vi "Kinesis-Microestruturacao-Circuits.vi"() -> ()   [LabVIEW 2014]
doc: "André Romero - 2017\nandretec@ifsc.usp.br"
uses:
  Basic-VIs/motorsGlobalVar.vi
  <vilib>/Instr/_visa.llb/VISA Configure Serial Port (Instr).vi
  C:/user-Lab/AndreTec/GITs/andretec/Thorlabs-Vector-Move/kinesisTec/Kinesis/Thorlabs.MotionControl.Controls.dll
  kinesisTec/Kinesis/Thorlabs.MotionControl.Controls.dll
panel:
  in  "Raio":dbl=0.01
  in  "Density":dbl=100.0
  in  "Adjust Motors":bool
  out "Process time":string="0:00:50"
  out "Progress %":dbl(slide) scale=0.0..100.0
  out "XY Graph":cluster{"Graph X":dbl[], "Graph Y":dbl[]}(graph)
  in  "Swap XY":bool
  out "stop cronometro":bool=TRUE
  in  "Stop Button":bool
  in  "Graph Y":dbl[](array[numeric])=[0.0, 0.0, 6.6674440298507465, 6.6674440298507465, 6.6674440298507465, 6.6674440298507465, 6.6674440298507465, 6.6674440298507465, 6.6674440298507465, 6.6674440298507465, 6.6674440298507465, 6.6674440298507465, 6.6674440298507465, 6.6674440298507465, 6.6674440298507465, 6.6674440298507465, 6.6674440298507465, 6.6674440298507465, 6.6674440298507465, 6.6674440298507465, 6.6674440298507465, 6.6674440298507465, 6.6674440298507465, 6.6674440298507465, 6.6674440298507465, 6.6674440298507465, 6.6674440298507465, 6.6674440298507465, 6.6674440298507465, 6.6674440298507465, 6.6674440298507465, 6.6674440298507465, 6.6674440298507465, 6.6674440298507465, 6.6674440298507465, 6.6674440298507465, 6.6674440298507465, 6.6674440298507465, 6.6674440298507465, 6.6674440298507465, 6.6674440298507465, 6.6674440298507465, 6.6674440298507465, 6.673128498134329, 6.673128498134329, 6.673128498134329, 6.673128498134329, 6.673128498134329, 6.687354244402985, 6.687354244402985, 6.687354244402985, 6.687354244402985, 6.687354244402985, 6.692543143656716, 6.692543143656716, 6.692543143656716, 6.692543143656716, 6.692543143656716, 6.692543143656716, 6.692543143656716, 6.692543143656716, 6.692543143656716, 6.692543143656716, 6.692543143656716, 6.692543143656716, 6.691522854477612, 6.691522854477612, 6.691522854477612, 6.691522854477612, 6.691522854477612, 6.680183069029851, 6.680183069029851, 6.680183069029851, 6.680183069029851, 6.680183069029851, 6.658640391791045, 6.658640391791045, 6.658640391791045, 6.658640391791045, 6.658640391791045, 6.644793610074627, 6.644793610074627, 6.644793610074627, 6.644793610074627, 6.644793610074627, 6.642490671641791, 6.642490671641791, 6.642490671641791, 6.642490671641791, 6.642490671641791, 6.642490671641791, 6.642490671641791, 6.642490671641791, 6.642490671641791, 6.642490671641791, 6.642490671641791, 6.642490671641791, 6.642490671641791, 6.642490671641791, 6.642490671641791, 6.647825326492537, 6.647825326492537, 6.647825326492537, 6.647825326492537, 6.647825326492537, 6.66543260261194, 6.66543260261194, 6.66543260261194, 6.66543260261194, 6.66543260261194, 6.685226212686567, 6.685226212686567, 6.685226212686567, 6.685226212686567, 6.685226212686567, 6.692484841417911, 6.692484841417911, 6.692484841417911, 6.692484841417911, 6.692484841417911, 6.692543143656716, 6.692543143656716, 6.692543143656716, 6.692543143656716, 6.692543143656716, 6.692543143656716, 6.692543143656716, 6.691464552238806, 6.691464552238806, 6.691464552238806, 6.691464552238806, 6.691464552238806, 6.679833255597015, 6.679833255597015, 6.679833255597015, 6.679833255597015, 6.679833255597015, 6.658057369402985, 6.658057369402985, 6.658057369402985, 6.658057369402985, 6.658057369402985, 6.644647854477612, 6.644647854477612, 6.644647854477612, 6.644647854477612, 6.644647854477612, 6.642548973880597, 6.642548973880597, 6.642548973880597, 6.642548973880597, 6.642548973880597, 6.642519822761194, 6.642519822761194, 6.642519822761194, 6.642519822761194, 6.642519822761194, 6.642519822761194, 6.642519822761194, 6.642519822761194, 6.643569263059701, 6.643569263059701, 6.643569263059701, 6.643569263059701, 6.643569263059701, 6.655521222014926, 6.655521222014926, 6.655521222014926, 6.655521222014926, 6.655521222014926, 6.677180503731344, 6.677180503731344, 6.677180503731344, 6.677180503731344, 6.677180503731344, 6.690531716417911, 6.690531716417911, 6.690531716417911, 6.690531716417911, 6.690531716417911, 6.692572294776119, 6.692572294776119, 6.692572294776119, 6.692572294776119, 6.692572294776119, 6.692572294776119, 6.692572294776119, 6.692572294776119, 6.692572294776119, 6.692572294776119, 6.692572294776119, 6.692572294776119, 6.691522854477612, 6.691522854477612, 6.691522854477612, 6.691522854477612, 6.691522854477612, 6.680008162313433, 6.680008162313433, 6.680008162313433, 6.680008162313433, 6.680008162313433, 6.668668376865671, 6.668668376865671, 6.668668376865671, 6.668668376865671, 6.668668376865671, 6.667502332089552, 6.667502332089552, 6.667502332089552, 6.667502332089552, 6.667502332089552, 6.667502332089552, 6.667502332089552, 6.667502332089552, 6.667502332089552, 6.667502332089552, 6.667502332089552, 6.667502332089552, 6.667531483208955, 6.667531483208955, 6.667531483208955, 6.667531483208955, 6.667531483208955, 6.667531483208955, 6.667531483208955, 6.667531483208955, 6.667531483208955, 6.667531483208955, 6.667531483208955, 6.667531483208955, 6.667531483208955, 6.667531483208955, 6.667531483208955, 6.667531483208955, 6.667531483208955, 6.667531483208955, 6.667531483208955, 6.667531483208955, 6.667531483208955, 6.667531483208955, 6.667531483208955, 6.667531483208955, 6.667531483208955, 6.667531483208955, 6.667531483208955, 6.667531483208955, 6.667531483208955, 6.667531483208955, 6.667531483208955, 6.667531483208955, 6.667531483208955, 6.667531483208955, 6.667531483208955, 6.667531483208955, 6.667531483208955, 6.6663945895522385, 6.6663945895522385, 6.6663945895522385, 6.6663945895522385, 6.6663945895522385, 6.662051072761194, 6.662051072761194, 6.662051072761194, 6.662051072761194, 6.662051072761194, 6.644035680970149, 6.644035680970149, 6.644035680970149, 6.644035680970149, 6.644035680970149, 6.606430736940299, 6.606430736940299, 6.606430736940299, 6.606430736940299, 6.606430736940299, 6.593924906716418, 6.593924906716418, 6.593924906716418, 6.593924906716418, 6.593924906716418, 6.574539412313433, 6.574539412313433, 6.574539412313433, 6.574539412313433, 6.574539412313433, 6.567484841417911, 6.567484841417911, 6.567484841417911, 6.567484841417911, 6.567484841417911, 6.567484841417911, 6.567484841417911, 6.567484841417911, 6.567484841417911, 6.567484841417911, 6.567484841417911, 6.567513992537314, 6.567513992537314, 6.567513992537314, 6.567513992537314, 6.567513992537314, 6.567513992537314, 6.567513992537314, 6.567513992537314, 6.567513992537314, 6.567513992537314, 6.567543143656716, 6.567543143656716, 6.567543143656716, 6.567543143656716, 6.567543143656716, 6.567543143656716, 6.567543143656716, 6.567543143656716, 6.567543143656716, 6.567543143656716, 6.567543143656716, 6.567543143656716, 6.567543143656716, 6.567543143656716, 6.567543143656716, 6.567543143656716, 6.567543143656716, 6.567543143656716, 6.567543143656716, 6.567543143656716, 6.567543143656716, 6.567543143656716, 6.567543143656716, 6.567543143656716, 6.567543143656716, 6.567543143656716, 6.567543143656716, 6.567543143656716, 6.567543143656716, 6.567543143656716, 6.567543143656716, 6.567543143656716, 6.567543143656716, 6.567543143656716, 6.567543143656716, 6.567543143656716, 6.567543143656716, 6.567543143656716, 6.567543143656716, 6.567543143656716, 6.567543143656716, 6.567543143656716, 6.567543143656716, 6.567543143656716, 6.567543143656716, 6.567543143656716, 6.567543143656716, 6.567543143656716, 6.567543143656716, 6.567543143656716, 6.567543143656716, 6.567543143656716, 6.567543143656716, 6.567543143656716, 6.5667852145522385, 6.5667852145522385, 6.5667852145522385, 6.5667852145522385, 6.5667852145522385, 6.555299673507463, 6.555299673507463, 6.555299673507463, 6.555299673507463, 6.555299673507463, 6.533523787313433, 6.533523787313433, 6.533523787313433, 6.533523787313433, 6.533523787313433, 6.525186567164179, 6.525186567164179, 6.525186567164179, 6.525186567164179, 6.525186567164179, 6.517490671641791, 6.517490671641791, 6.517490671641791, 6.517490671641791, 6.517490671641791, 6.517490671641791, 6.517490671641791, 6.517490671641791, 6.517490671641791, 6.517490671641791, 6.517519822761194, 6.517519822761194, 6.517519822761194, 6.517519822761194, 6.517519822761194, 6.517519822761194, 6.517519822761194, 6.517519822761194, 6.517519822761194, 6.517519822761194, 6.517548973880597, 6.517548973880597, 6.517548973880597, 6.517548973880597, 6.517548973880597, 6.517548973880597, 6.517548973880597, 6.517548973880597, 6.517548973880597, 6.517548973880597, 6.517548973880597, 6.517548973880597, 6.517548973880597, 6.517548973880597, 6.517548973880597, 6.517548973880597, 6.517548973880597, 6.517548973880597, 6.517548973880597, 6.517548973880597, 6.517548973880597, 6.517548973880597, 6.517548973880597, 6.517548973880597, 6.517548973880597, 6.517548973880597, 6.517548973880597, 6.517548973880597, 6.517548973880597, 6.517548973880597, 6.517548973880597, 6.517548973880597, 6.517548973880597, 6.517548973880597, 6.517548973880597, 6.517548973880597, 6.517548973880597, 6.517548973880597, 6.517548973880597, 6.517548973880597, 6.517548973880597, 6.517548973880597, 6.517548973880597, 6.517548973880597, 6.517548973880597, 6.517548973880597, 6.517548973880597, 6.517548973880597, 6.517548973880597, 6.517548973880597, 6.517548973880597, 6.517548973880597, 6.517548973880597, 6.517548973880597, 6.517548973880597, 6.517548973880597, 6.517548973880597, 6.517548973880597, 6.517548973880597, 6.517548973880597, 6.516674440298507, 6.516674440298507, 6.516674440298507, 6.516674440298507, 6.516674440298507, 6.504897388059701, 6.504897388059701, 6.504897388059701, 6.504897388059701, 6.504897388059701, 6.481926305970149, 6.481926305970149, 6.481926305970149, 6.481926305970149, 6.481926305970149, 6.456943796641791, 6.456943796641791, 6.456943796641791, 6.456943796641791, 6.456943796641791, 6.4330690298507465, 6.4330690298507465, 6.4330690298507465, 6.4330690298507465, 6.4330690298507465, 6.419717817164179, 6.419717817164179, 6.419717817164179, 6.419717817164179, 6.419717817164179, 6.417473180970149, 6.417473180970149, 6.417473180970149, 6.417473180970149, 6.417473180970149, 6.417473180970149]
  in  "Graph X":dbl[](array[numeric])=[0.0, 0.0, 3.605935167910448, 3.605935167910448, 3.605935167910448, 3.605935167910448, 3.605935167910448, 3.609987173507463, 3.609987173507463, 3.609987173507463, 3.609987173507463, 3.609987173507463, 3.627157182835821, 3.627157182835821, 3.627157182835821, 3.627157182835821, 3.627157182835821, 3.6520813899253732, 3.6520813899253732, 3.6520813899253732, 3.6520813899253732, 3.6520813899253732, 3.6770930503731343, 3.6770930503731343, 3.6770930503731343, 3.6770930503731343, 3.6770930503731343, 3.697323927238806, 3.697323927238806, 3.697323927238806, 3.697323927238806, 3.697323927238806, 3.705311333955224, 3.705311333955224, 3.705311333955224, 3.705311333955224, 3.705311333955224, 3.705311333955224, 3.705311333955224, 3.705311333955224, 3.705311333955224, 3.705311333955224, 3.705311333955224, 3.7063024720149254, 3.7063024720149254, 3.7063024720149254, 3.7063024720149254, 3.7063024720149254, 3.7175839552238807, 3.7175839552238807, 3.7175839552238807, 3.7175839552238807, 3.7175839552238807, 3.7291861007462686, 3.7291861007462686, 3.7291861007462686, 3.7291861007462686, 3.7291861007462686, 3.7303521455223883, 3.7303521455223883, 3.7303521455223883, 3.7303521455223883, 3.7303521455223883, 3.7303521455223883, 3.7303521455223883, 3.7303521455223883, 3.7303521455223883, 3.7303521455223883, 3.7303521455223883, 3.7303521455223883, 3.7366779384328357, 3.7366779384328357, 3.7366779384328357, 3.7366779384328357, 3.7366779384328357, 3.7554221082089554, 3.7554221082089554, 3.7554221082089554, 3.7554221082089554, 3.7554221082089554, 3.774137126865672, 3.774137126865672, 3.774137126865672, 3.774137126865672, 3.774137126865672, 3.7803463152985075, 3.7803463152985075, 3.7803463152985075, 3.7803463152985075, 3.7803463152985075, 3.7803463152985075, 3.7803463152985075, 3.7803463152985075, 3.7803463152985075, 3.7803463152985075, 3.7803463152985075, 3.7803463152985075, 3.7803463152985075, 3.7803463152985075, 3.7803463152985075, 3.781803871268657, 3.781803871268657, 3.781803871268657, 3.781803871268657, 3.781803871268657, 3.7941930970149254, 3.7941930970149254, 3.7941930970149254, 3.7941930970149254, 3.7941930970149254, 3.816027285447761, 3.816027285447761, 3.816027285447761, 3.816027285447761, 3.816027285447761, 3.828678871268657, 3.828678871268657, 3.828678871268657, 3.828678871268657, 3.828678871268657, 3.8303404850746268, 3.8303404850746268, 3.8303404850746268, 3.8303404850746268, 3.8303404850746268, 3.8303404850746268, 3.8303404850746268, 3.8303404850746268, 3.8303404850746268, 3.8303404850746268, 3.8303404850746268, 3.8303404850746268, 3.8368703358208953, 3.8368703358208953, 3.8368703358208953, 3.8368703358208953, 3.8368703358208953, 3.8447994402985075, 3.8447994402985075, 3.8447994402985075, 3.8447994402985075, 3.8447994402985075, 3.866633628731343, 3.866633628731343, 3.866633628731343, 3.866633628731343, 3.866633628731343, 3.8803346548507465, 3.8803346548507465, 3.8803346548507465, 3.8803346548507465, 3.8803346548507465, 3.8803346548507465, 3.8803346548507465, 3.8803346548507465, 3.8803346548507465, 3.8803346548507465, 3.8803346548507465, 3.8803346548507465, 3.8803346548507465, 3.8803346548507465, 3.8803346548507465, 3.8803346548507465, 3.8803346548507465, 3.8803346548507465, 3.886631296641791, 3.886631296641791, 3.886631296641791, 3.886631296641791, 3.886631296641791, 3.9054046175373136, 3.9054046175373136, 3.9054046175373136, 3.9054046175373136, 3.9054046175373136, 3.92411963619403, 3.92411963619403, 3.92411963619403, 3.92411963619403, 3.92411963619403, 3.9303288246268657, 3.9303288246268657, 3.9303288246268657, 3.9303288246268657, 3.9303288246268657, 3.9303288246268657, 3.9303288246268657, 3.9303288246268657, 3.9303288246268657, 3.9303288246268657, 3.9303288246268657, 3.9303288246268657, 3.9303288246268657, 3.9303288246268657, 3.9303288246268657, 3.9303288246268657, 3.9303288246268657, 3.936800373134328, 3.936800373134328, 3.936800373134328, 3.936800373134328, 3.936800373134328, 3.9445545708955225, 3.9445545708955225, 3.9445545708955225, 3.9445545708955225, 3.9445545708955225, 3.95536963619403, 3.95536963619403, 3.95536963619403, 3.95536963619403, 3.95536963619403, 3.95536963619403, 3.95536963619403, 3.95536963619403, 3.95536963619403, 3.95536963619403, 3.95536963619403, 3.95536963619403, 3.956652285447761, 3.956652285447761, 3.956652285447761, 3.956652285447761, 3.956652285447761, 3.961141557835821, 3.961141557835821, 3.961141557835821, 3.961141557835821, 3.961141557835821, 3.9795067630597014, 3.9795067630597014, 3.9795067630597014, 3.9795067630597014, 3.9795067630597014, 4.004518423507463, 4.004518423507463, 4.004518423507463, 4.004518423507463, 4.004518423507463, 4.0406366604477615, 4.0406366604477615, 4.0406366604477615, 4.0406366604477615, 4.0406366604477615, 4.048624067164179, 4.048624067164179, 4.048624067164179, 4.048624067164179, 4.048624067164179, 4.0553579757462686, 4.0553579757462686, 4.0553579757462686, 4.0553579757462686, 4.0553579757462686, 4.0553579757462686, 4.0553579757462686, 4.055387126865671, 4.055387126865671, 4.055387126865671, 4.055387126865671, 4.055387126865671, 4.055387126865671, 4.055387126865671, 4.055387126865671, 4.055387126865671, 4.055387126865671, 4.0553579757462686, 4.0553579757462686, 4.0553579757462686, 4.0553579757462686, 4.0553579757462686, 4.0553579757462686, 4.0553579757462686, 4.0553579757462686, 4.0553579757462686, 4.0553579757462686, 4.0553579757462686, 4.0553579757462686, 4.0553579757462686, 4.0553579757462686, 4.0553579757462686, 4.0553579757462686, 4.0553579757462686, 4.0553579757462686, 4.0553579757462686, 4.0553579757462686, 4.0553579757462686, 4.0553579757462686, 4.0553579757462686, 4.0553579757462686, 4.0553579757462686, 4.0553579757462686, 4.0553579757462686, 4.0553579757462686, 4.0553579757462686, 4.0553579757462686, 4.0553579757462686, 4.061800373134329, 4.061800373134329, 4.061800373134329, 4.061800373134329, 4.061800373134329, 4.06972947761194, 4.06972947761194, 4.06972947761194, 4.06972947761194, 4.06972947761194, 4.091534514925373, 4.091534514925373, 4.091534514925373, 4.091534514925373, 4.091534514925373, 4.105352145522388, 4.105352145522388, 4.105352145522388, 4.105352145522388, 4.105352145522388, 4.105381296641791, 4.105381296641791, 4.105381296641791, 4.105381296641791, 4.105381296641791, 4.105381296641791, 4.105381296641791, 4.1050897854477615, 4.1050897854477615, 4.1050897854477615, 4.1050897854477615, 4.1050897854477615, 4.0951784048507465, 4.0951784048507465, 4.0951784048507465, 4.0951784048507465, 4.0951784048507465, 4.073489972014926, 4.073489972014926, 4.073489972014926, 4.073489972014926, 4.073489972014926, 4.060954990671642, 4.060954990671642, 4.060954990671642, 4.060954990671642, 4.060954990671642, 4.023874766791045, 4.023874766791045, 4.023874766791045, 4.023874766791045, 4.023874766791045, 4.008687033582089, 4.008687033582089, 4.008687033582089, 4.008687033582089, 4.008687033582089, 4.005363805970149, 4.005363805970149, 4.005363805970149, 4.005363805970149, 4.005363805970149, 4.005363805970149, 4.005363805970149, 4.005363805970149, 4.005363805970149, 4.005363805970149, 4.005363805970149, 4.005363805970149, 4.005363805970149, 4.005363805970149, 4.005363805970149, 4.005363805970149, 4.005363805970149, 4.005392957089552, 4.005392957089552, 4.005392957089552, 4.005392957089552, 4.005392957089552, 4.005392957089552, 4.005392957089552, 4.005392957089552, 4.005392957089552, 4.005392957089552, 4.005392957089552, 4.005392957089552, 4.005392957089552, 4.005392957089552, 4.005392957089552, 4.005392957089552, 4.005392957089552, 4.005392957089552, 4.005392957089552, 4.005392957089552, 4.011631296641791, 4.011631296641791, 4.011631296641791, 4.011631296641791, 4.011631296641791, 4.019472947761194, 4.019472947761194, 4.019472947761194, 4.019472947761194, 4.019472947761194, 4.042852145522388, 4.042852145522388, 4.042852145522388, 4.042852145522388, 4.042852145522388, 4.080398787313433, 4.080398787313433, 4.080398787313433, 4.080398787313433, 4.080398787313433, 4.099113805970149, 4.099113805970149, 4.099113805970149, 4.099113805970149, 4.099113805970149, 4.103777985074627, 4.103777985074627, 4.103777985074627, 4.103777985074627, 4.103777985074627, 4.105410447761194, 4.105410447761194, 4.105410447761194, 4.105410447761194, 4.105410447761194, 4.105410447761194, 4.105410447761194, 4.105410447761194, 4.105381296641791, 4.105381296641791, 4.105381296641791, 4.105381296641791, 4.105381296641791, 4.098297574626866, 4.098297574626866, 4.098297574626866, 4.098297574626866, 4.098297574626866, 4.089989505597015, 4.089989505597015, 4.089989505597015, 4.089989505597015, 4.089989505597015, 4.06083838619403, 4.06083838619403, 4.06083838619403, 4.06083838619403, 4.06083838619403, 4.0553579757462686, 4.0553579757462686, 4.0553579757462686, 4.0553579757462686, 4.0553579757462686, 4.0553579757462686, 4.0553579757462686, 4.0553579757462686, 4.0553579757462686, 4.0553579757462686, 4.0553579757462686, 4.0553579757462686, 4.055387126865671, 4.055387126865671, 4.055387126865671, 4.055387126865671, 4.055387126865671, 4.055416277985074, 4.055416277985074, 4.055416277985074, 4.055416277985074, 4.055416277985074, 4.055416277985074, 4.055416277985074, 4.055416277985074, 4.055416277985074, 4.055416277985074, 4.055416277985074, 4.055416277985074, 4.055416277985074, 4.055416277985074, 4.055416277985074, 4.055416277985074, 4.055416277985074, 4.055416277985074, 4.055416277985074, 4.055416277985074, 4.055416277985074, 4.055416277985074, 4.055416277985074, 4.055416277985074, 4.055416277985074, 4.055416277985074, 4.055416277985074, 4.055416277985074, 4.055416277985074, 4.055416277985074, 4.055416277985074]
  out "GetPOS Y":dbl=6.417473180970149 format="%_6f"
  out "GetPOS X":dbl=4.055416277985074 format="%#_6f"
  out ".NET Refnum out 2":refnum<k24>
  out ".NET Refnum out 1":refnum<k24>
  out "Motor 2":bool
  out "Motor 1":bool
  in  "Acceleration (mm/s)":dbl=0.05
  in  "Iniciar":bool
  in  "Velocity (mm/s)":sgl=0.05
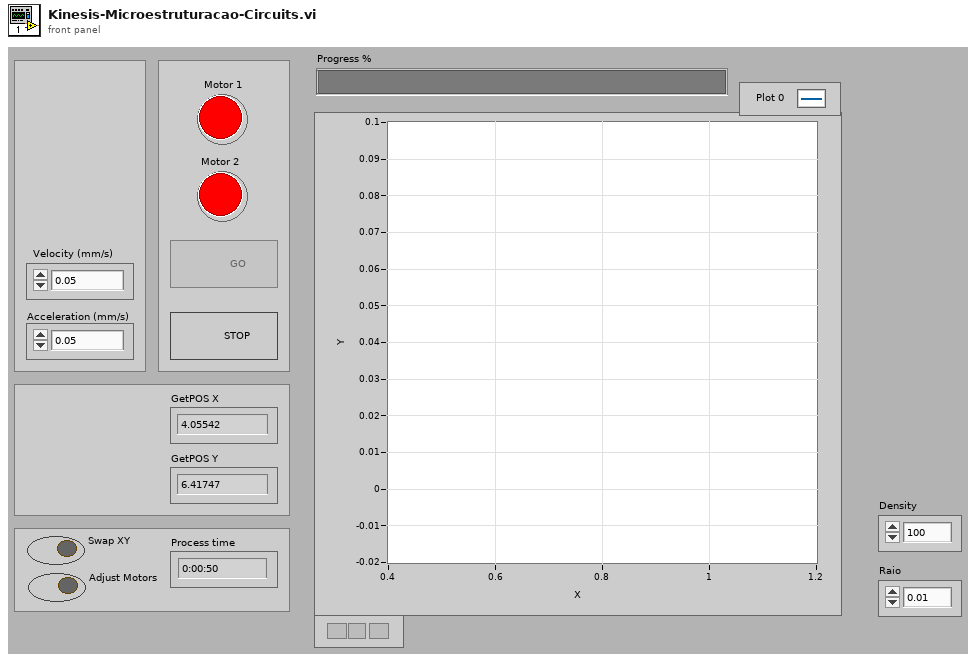
[diagram p1: front panel]
types:
  T1 = enum8{"Enabled", "Disabled", "Disabled and Grayed Out"}
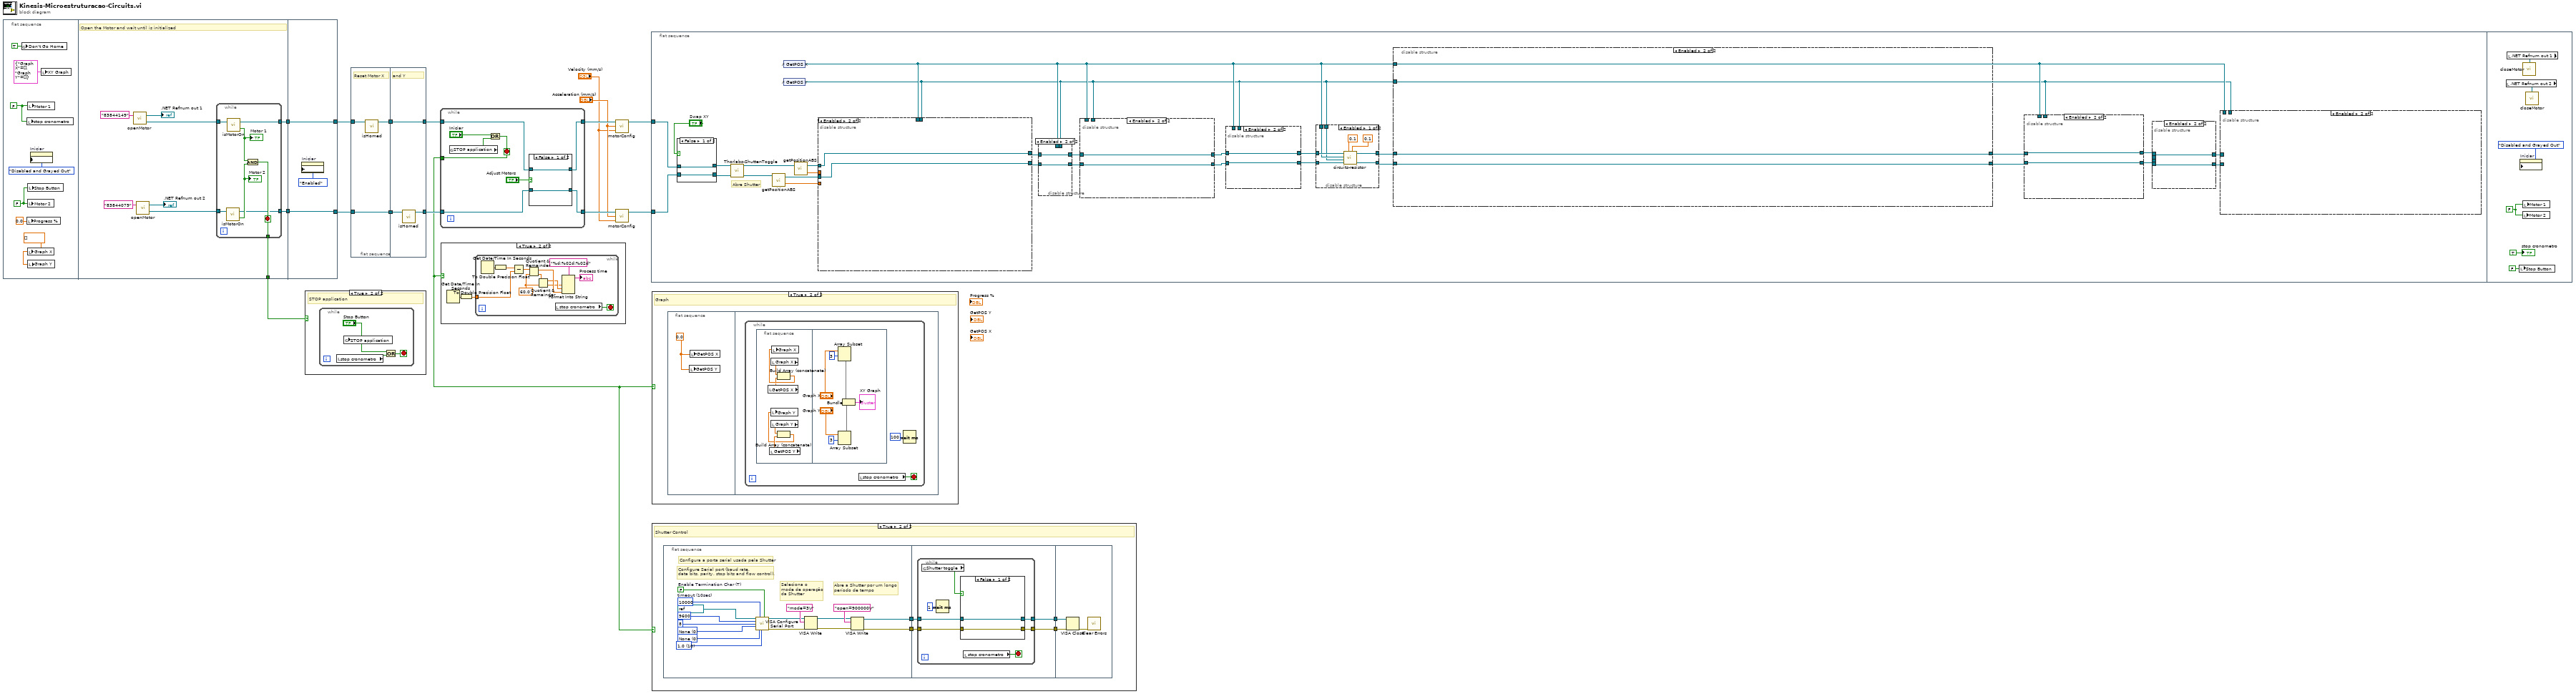
[diagram p0: block diagram]
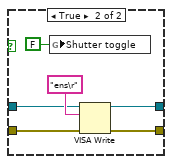
[diagram p3: hidden frame]
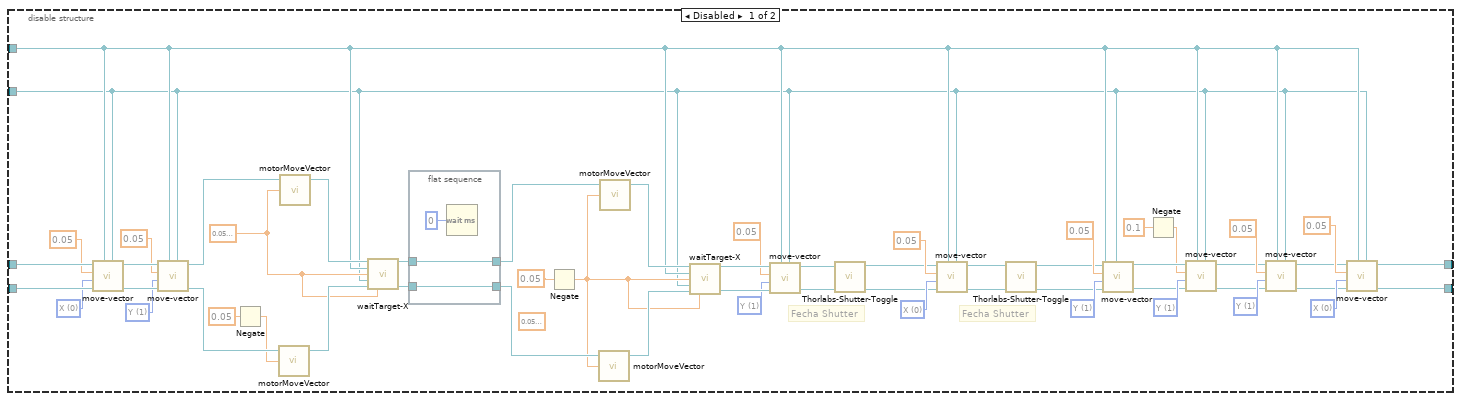
[diagram p6: hidden frame]
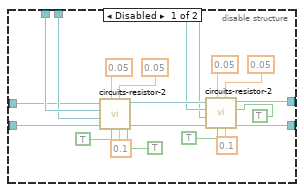
[diagram p7: hidden frame]
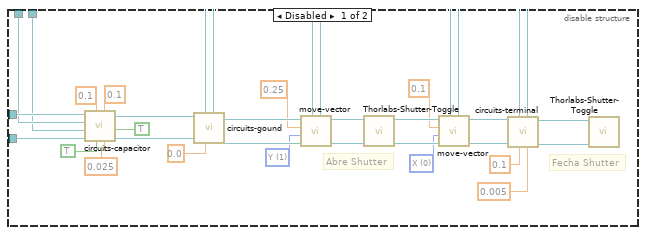
[diagram p8: hidden frame]
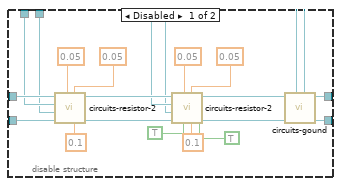
[diagram p9: hidden frame]
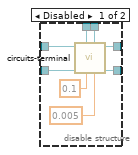
[diagram p10: hidden frame]
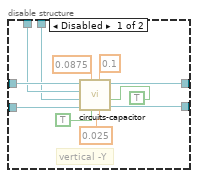
[diagram p12: hidden frame]
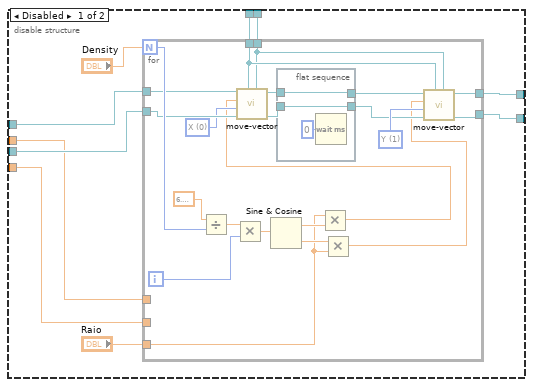
[diagram p13: hidden frame]
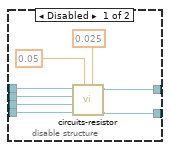
[diagram p14: hidden frame]
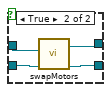
[diagram p15: hidden frame]
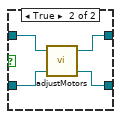
[diagram p17: hidden frame]
diagram:
  n1 = flat-sequence {
    tunnel: [w32] -> w4
    tunnel: [w31] -> w3
    tunnel: [w30] -> w2
    tunnel: [w41] -> w7
    tunnel: [w42] -> w8
    tunnel: w4 -> [w42]
    tunnel: w3 -> [w41]
    frame #0 {
      w19 = dbl[] [] ("Graph Y")
      w22 = FALSE ("Motor3\nLigado")
      w23 = FALSE
      n2 = global write "motorsGlobalVar.vi" "Don't Go Home"(TRUE ("Don't Go Home")) -> ()
      n3 = local write "stop cronometro"(w23) -> ()
      n4 = local write "Progress %"(0.0 ("Progress %")) -> ()
      n5 = local write "Motor 2"(w22) -> ()
      n6 = local write "Graph X"(w19) -> ()
      n7 = local write "Motor 1"(w23) -> ()
      n8 = local write "Stop Button"(w22) -> ()
      n9 = local write "Graph Y"(w19) -> ()
      n10 = property on="Iniciar" class="Bool (strict)"("DisabledEnum"=T1."Disabled and Grayed Out" ("Disabled")) -> ()  [unwired: 2 in, 2 out]
      n11 = local write "XY Graph"(cluster{"Graph X":dbl[], "Graph Y":dbl[]} {"Graph X"=[], "Graph Y"=[]} ("XY Graph")) -> ()
    }
    frame #1 {
      # "Open the Motor and wait until is initialized"
      n12 = call "openMotor.vi"("S/N Motor"="83844149") -> ("Device"=w28:refnum<k24>, ".NET Refnum out"=→".NET Refnum out 1":refnum<k24>)  [unwired: 1 in]
      n13 = call "openMotor.vi"("S/N Motor"="83844079") -> ("Device"=w29:refnum<k24>, ".NET Refnum out"=→".NET Refnum out 2":refnum<k24>)  [unwired: 1 in]
      n14 = while {
        tunnel: w28 -> [w37]
        tunnel: w29 -> [w36]
        tunnel: [w34] -> w32
        tunnel: [w33] -> w31
        tunnel: [w35] -> w30
        stop <- w35 stop-if-true
        n15 = call "isMotorOn.vi"("Device"=w36) -> ("isConnected"=w38:bool, "Device out"=w33:refnum<k24>)  [unwired: 1 in]
        "Motor 2" <- w38
        n16 = call "isMotorOn.vi"("Device"=w37) -> ("isConnected"=w39:bool, "Device out"=w34:refnum<k24>)  [unwired: 1 in]
        "Motor 1" <- w39
        n17 = And(x=w39, y=w38) -> (x .and. y?=w35:bool)
      }
    }
    frame #2 {
      n18 = property on="Iniciar" class="Bool (strict)"("DisabledEnum"=T1."Enabled" ("Disabled")) -> ()  [unwired: 2 in, 2 out]
    }
  }
  n19 = case shown="True" w2 {
    frame False {
    }
    frame True {
      # "STOP application"
      n20 = while {
        stop <- w44 stop-if-true
        n21 = local read "stop cronometro"() -> (w43:bool)
        n22 = global write "motorsGlobalVar.vi" "STOP application"("Stop Button") -> ()
        n23 = Or(x="Stop Button", y=w43) -> (x .or. y?=w44:bool)
      }
    }
  }
  n24 = flat-sequence {
    tunnel: w8 -> [w48]
    tunnel: w7 -> [w46]
    tunnel: [w47] -> w6
    tunnel: [w46] -> w5
    tunnel: [w51] -> w10
    tunnel: [w50] -> w9
    tunnel: w6 -> [w51]
    tunnel: w5 -> [w49]
    frame #0 {
      # "Reset Motor X"
      n25 = call "isHomed.vi"("Device in"=w48) -> ("Device out"=w47:refnum<k24>)  [unwired: 4 in]
    }
    frame #1 {
      # "and Y"
      n26 = call "isHomed.vi"("Device in"=w49) -> ("Device out"=w50:refnum<k24>)  [unwired: 4 in]
    }
  }
  n27 = while {
    tunnel: [w59] -> w1
    tunnel: w10 -> [w54]
    tunnel: w9 -> [w55]
    tunnel: [w53] -> w16
    tunnel: [w52] -> w15
    stop <- w59 stop-if-true
    n28 = global read "motorsGlobalVar.vi" "STOP application"() -> (w57:bool)
    n29 = Or(x="Iniciar", y=w57) -> (x .or. y?=w59:bool)
    n30 = case shown="False" "Adjust Motors" {
      tunnel: w55 -> [w60 w65]
      tunnel: w54 -> [w61 w64]
      tunnel: [w61 w63] -> w53
      tunnel: [w60 w62] -> w52
      frame False {
      }
      frame True {
        n31 = call "adjustMotors.vi"("Device 2"=w65, "Device 1"=w64) -> ("Device out 2"=w62:refnum<k24>, "Device out 1"=w63:refnum<k24>)  [unwired: 2 in]
      }
    }
  }
  n32 = case shown="True" w1 {
    frame False {
    }
    frame True {
      n33 = Get Date/Time In Seconds() -> (seconds since 1Jan1904=w67:timestamp)
      n34 = To Double Precision Float(number=w67) -> (double precision float=w66:dbl)
      n35 = while {
        tunnel: w66 -> [w71]
        stop <- w79 stop-if-true
        w76 = 60.0 ("y")
        n36 = Get Date/Time In Seconds() -> (seconds since 1Jan1904=w78:timestamp)
        n37 = To Double Precision Float(number=w78) -> (double precision float=w72:dbl)
        n38 = Subtract(x=w72, y=w71) -> (x-y=w70:dbl)
        n39 = Quotient & Remainder(x=w70, y=w76) -> (x-y*floor(x/y)=w75:dbl, floor(x/y)=w77:dbl)
        n40 = Quotient & Remainder(x=w77, y=w76) -> (x-y*floor(x/y)=w74:dbl, floor(x/y)=w73:dbl)
        n41 = local read "stop cronometro"() -> (w79:bool)
        n42 = Format Into String(format string="%d:%02d:%02d", w73, w74, w75) -> (resulting string=→"Process time":string)  [unwired: 2 in, 1 out]
      }
    }
  }
  n43 = call "motorConfig.vi"("Velocity"="Velocity (mm/s)", "Acceleration"="Acceleration (mm/s)", "Device in"=w16) -> ("Device out"=w12:refnum<k24>)  [unwired: 2 in]
  n44 = call "motorConfig.vi"("Velocity"="Velocity (mm/s)", "Acceleration"="Acceleration (mm/s)", "Device in"=w15) -> ("Device out"=w11:refnum<k24>)  [unwired: 2 in]
  n45 = flat-sequence {
    tunnel: w12 -> [w108]
    tunnel: w11 -> [w107]
    frame #0 {
      # "Abre Shutter"
      n46 = case shown="False" "Swap XY" {
        tunnel: w108 -> [w319 w323]
        tunnel: w107 -> [w318 w322]
        tunnel: [w319 w321] -> w103
        tunnel: [w318 w320] -> w102
        frame False {
        }
        frame True {
          n47 = call "swapMotors.vi"("Device 2"=w322, "Device 1"=w323) -> ("Device out 1"=w320:refnum<k24>, "Device out 2"=w321:refnum<k24>)  [unwired: 2 in, 2 out]
        }
      }
      n48 = call "Thorlabs-Shutter-Toggle.vi"("Device in Y"=w102, "Device in X"=w103) -> ("Device out Y"=w99:refnum<k24>, "Device out X"=w101:refnum<k24>)  [unwired: 8 in]
      n49 = call "getPositionABS.vi"("Device"=w99) -> ("GetPOS"=w96:dbl, "Device out"=w98:refnum<k24>)  [unwired: 1 in]
      n50 = control-ref of="GetPOS X"() -> (w83:refnum<vi>)
      n51 = control-ref of="GetPOS Y"() -> (w82:refnum<vi>)
      n52 = call "getPositionABS.vi"("Device"=w101) -> ("GetPOS"=w97:dbl, "Device out"=w100:refnum<k24>)  [unwired: 1 in]
      n53 = disable-structure shown="Enabled" {
        disable-tunnel: w100 -> [w278 w307]
        disable-tunnel: w98 -> [w277 w306]
        disable-tunnel: w97 -> [w276 _]
        disable-tunnel: w96 -> [w275 _]
        disable-tunnel: w83 -> [w274 _]
        disable-tunnel: w82 -> [w273 _]
        disable-tunnel: [w272 w307] -> w91
        disable-tunnel: [w271 w306] -> w90
        frame Disabled {
          n54 = for {
            N: "Density" -> [w297]
            tunnel: w276 -> [_]
            tunnel: w275 -> [_]
            tunnel: "Raio" -> [w295]
            tunnel: w278 -> [w294]
            tunnel: w277 -> [w293]
            tunnel: w274 -> [w288]
            tunnel: w273 -> [w287]
            tunnel: [w290] -> w272
            tunnel: [w289] -> w271
            i -> [w296]
            w291 = u16 1 items=["X", "Y"] ("X-Y")
            w292 = u16 0 items=["X", "Y"] ("X-Y")
            n55 = Divide(x=6.283185307179586, y=w297) -> (x/y=w302:dbl)
            n56 = Multiply(x=w302, y=w296) -> (x*y=w301:dbl)
            n57 = Sine & Cosine(0:w301) -> (1:w300:dbl, 2:w299:dbl)
            n58 = flat-sequence {
              tunnel: w286 -> [w305]
              tunnel: [w305] -> w283
              tunnel: w285 -> [w304]
              tunnel: [w304] -> w284
              frame #0 {
                n59 = Wait (ms)(milliseconds to wait=u32 0) -> ()  [unwired: 1 out]
              }
            }
            n60 = Multiply(x=w295, y=w300) -> (x*y=w282:dbl)
            n61 = call "move-vector.vi"("GetPOS Y"=w287, "GetPOS X"=w288, "Device in Y"=w293, "X-Y"=w292, "Distance"=w282, "Device in X"=w294) -> ("Device out Y"=w285:refnum<k24>, "Device out X"=w286:refnum<k24>)  [unwired: 4 in]
            n62 = Multiply(x=w299, y=w295) -> (x*y=w281:dbl)
            n63 = call "move-vector.vi"("GetPOS Y"=w287, "GetPOS X"=w288, "Device in Y"=w284, "X-Y"=w291, "Distance"=w281, "Device in X"=w283) -> ("Device out Y"=w289:refnum<k24>, "Device out X"=w290:refnum<k24>)  [unwired: 4 in]
          }
        }
        frame Enabled {
        }
      }
      n64 = disable-structure shown="Enabled" {
        disable-tunnel: w91 -> [w243 w247]
        disable-tunnel: w90 -> [w242 w246]
        disable-tunnel: [w241 w247] -> w89
        disable-tunnel: w83 -> [w240 _]
        disable-tunnel: w82 -> [w239 _]
        disable-tunnel: [w238 w246] -> w86
        frame Disabled {
          n65 = call "circuits-terminal.vi"("Density"=0.005, "GetPOS Y"=w239, "Diension"=0.1, "GetPOS X"=w240, "Device in Y"=w242, "Device in X"=w243) -> ("Device out Y"=w238:refnum<k24>, "Device out X"=w241:refnum<k24>)  [unwired: 4 in]
        }
        frame Enabled {
        }
      }
      n66 = disable-structure shown="Enabled" {
        disable-tunnel: w89 -> [w232 w237]
        disable-tunnel: w83 -> [w222 _]
        disable-tunnel: w82 -> [w221 _]
        disable-tunnel: [w220 w237] -> w88
        disable-tunnel: [w219 w236] -> w87
        disable-tunnel: w86 -> [w218 w236]
        frame Disabled {
          n67 = call "circuits-resistor-2.vi"("L3"=0.1, "L2"=0.05, "L1"=0.05, "Device in Y"=w218, "GetPOS Y"=w221, "GetPOS X"=w222, "Device in X"=w232) -> ("Device out Y"=w227:refnum<k24>, "Device out X"=w228:refnum<k24>)  [unwired: 3 in]
          n68 = call "circuits-resistor-2.vi"("Invert X"=TRUE, "L3"=0.1, "L2"=0.05, "Swap-XY"=TRUE, "L1"=0.05, "Device in Y"=w227, "GetPOS Y"=w221, "GetPOS X"=w222, "Device in X"=w228) -> ("Device out Y"=w223:refnum<k24>, "Device out X"=w224:refnum<k24>)  [unwired: 1 in]
          n69 = call "circuits-gound.vi"("GetPOS Y"=w221, "GetPOS X"=w222, "Device in Y"=w223, "Device in X"=w224) -> ("Device out Y"=w219:refnum<k24>, "Device out X"=w220:refnum<k24>)  [unwired: 6 in]
        }
        frame Enabled {
        }
      }
      n70 = disable-structure shown="Enabled" {
        disable-tunnel: w88 -> [w264 w270]
        disable-tunnel: [w263 w270] -> w95
        disable-tunnel: [w262 w269] -> w94
        disable-tunnel: w87 -> [w261 w269]
        disable-tunnel: w83 -> [w260 _]
        disable-tunnel: w82 -> [w259 _]
        frame Disabled {
          # "vertical -Y"
          n71 = call "circuits-capacitor.vi"("Invert Y"=TRUE, "L2"=0.025, "L3"=0.1, "Swap-XY"=TRUE, "L1"=0.0875, "Device in Y"=w261, "GetPOS Y"=w259, "GetPOS X"=w260, "Device in X"=w264) -> ("Device out Y"=w262:refnum<k24>, "Device out X"=w263:refnum<k24>)  [unwired: 1 in]
        }
        frame Enabled {
        }
      }
      n72 = disable-structure shown="Enabled" {
        disable-tunnel: w95 -> [w253 w257]
        disable-tunnel: w94 -> [w252 w256]
        disable-tunnel: [w251 w257] -> w85
        disable-tunnel: [w250 w256] -> w84
        disable-tunnel: w83 -> [w249 _]
        disable-tunnel: w82 -> [w248 _]
        frame Enabled {
          n73 = call "circuits-resistor.vi"("L2"=0.1, "L1"=0.1, "Device in Y"=w252, "GetPOS Y"=w248, "GetPOS X"=w249, "Device in X"=w253) -> ("Device out Y"=w250:refnum<k24>, "Device out X"=w251:refnum<k24>)  [unwired: 4 in]
        }
        frame Disabled {
        }
      }
      n74 = disable-structure shown="Enabled" {
        disable-tunnel: w85 -> [w159 w169]
        disable-tunnel: w84 -> [w158 w168]
        disable-tunnel: w83 -> [w112 _]
        disable-tunnel: w82 -> [w111 _]
        disable-tunnel: [w110 w169] -> w81
        disable-tunnel: [w109 w168] -> w80
        frame Disabled {
          w115 = u16 0 items=["X", "Y"] ("X-Y")
          w120 = u16 1 items=["X", "Y"] ("X-Y")
          w125 = u16 1 items=["X", "Y"] ("X-Y")
          w129 = u16 1 items=["X", "Y"] ("X-Y")
          w134 = u16 0 items=["X", "Y"] ("X-Y")
          w140 = u16 1 items=["X", "Y"] ("X-Y")
          w153 = u16 1 items=["X", "Y"] ("X-Y")
          w156 = u16 0 items=["X", "Y"] ("X-Y")
          (unwired) sgl 0.05 ("Distance")
          w143 = sgl 0.05 ("Distance")
          # "Fecha Shutter"
          # "Fecha Shutter"
          n75 = call "move-vector.vi"("GetPOS Y"=w111, "GetPOS X"=w112, "Device in Y"=w158, "X-Y"=w156, "Distance"=0.05, "Device in X"=w159) -> ("Device out Y"=w154:refnum<k24>, "Device out X"=w155:refnum<k24>)  [unwired: 4 in]
          n76 = call "move-vector.vi"("GetPOS Y"=w111, "GetPOS X"=w112, "Device in Y"=w154, "X-Y"=w153, "Distance"=0.05, "Device in X"=w155) -> ("Device out Y"=w150:refnum<k24>, "Device out X"=w151:refnum<k24>)  [unwired: 4 in]
          n77 = Negate(x=0.05) -> (-x=w148:dbl)
          n78 = call "motorMoveVector.vi"("Distance"=w148, "Device in"=w150) -> ("Device out"=w164:refnum<k24>)  [unwired: 3 in]
          n79 = call "motorMoveVector.vi"("Distance"=w143, "Device in"=w151) -> ("Device out"=w163:refnum<k24>)  [unwired: 3 in]
          n80 = call "waitTarget-X.vi"("Device in X"=w163, "GetPOS X"=w112, "Position X"=w143, "GetPOS Y"=w111, "Device in Y"=w164, "Position Y"=w143) -> ("Device out X"=w147:refnum<k24>, "Device out Y"=w146:refnum<k24>)  [unwired: 6 in, 2 out]
          n81 = flat-sequence {
            tunnel: w147 -> [w167]
            tunnel: w146 -> [w166]
            tunnel: [w167] -> w145
            tunnel: [w166] -> w144
            frame #0 {
              n82 = Wait (ms)(milliseconds to wait=u32 0) -> ()  [unwired: 1 out]
            }
          }
          n83 = Negate(x=0.05) -> (-x=w139:dbl)
          n84 = call "motorMoveVector.vi"("Distance"=w139, "Device in"=w144) -> ("Device out"=w162:refnum<k24>)  [unwired: 3 in]
          n85 = call "motorMoveVector.vi"("Distance"=w139, "Device in"=w145) -> ("Device out"=w161:refnum<k24>)  [unwired: 3 in]
          n86 = call "waitTarget-X.vi"("Device in X"=w161, "GetPOS X"=w112, "Position X"=w139, "GetPOS Y"=w111, "Device in Y"=w162, "Position Y"=w139) -> ("Device out X"=w142:refnum<k24>, "Device out Y"=w141:refnum<k24>)  [unwired: 6 in, 2 out]
          n87 = call "move-vector.vi"("GetPOS Y"=w111, "GetPOS X"=w112, "Device in Y"=w141, "X-Y"=w140, "Distance"=0.05, "Device in X"=w142) -> ("Device out Y"=w136:refnum<k24>, "Device out X"=w137:refnum<k24>)  [unwired: 4 in]
          n88 = call "Thorlabs-Shutter-Toggle.vi"("Device in Y"=w136, "Device in X"=w137) -> ("Device out Y"=w132:refnum<k24>, "Device out X"=w133:refnum<k24>)  [unwired: 8 in]
          n89 = call "move-vector.vi"("GetPOS Y"=w111, "GetPOS X"=w112, "Device in Y"=w132, "X-Y"=w134, "Distance"=0.05, "Device in X"=w133) -> ("Device out Y"=w130:refnum<k24>, "Device out X"=w131:refnum<k24>)  [unwired: 4 in]
          n90 = call "Thorlabs-Shutter-Toggle.vi"("Device in Y"=w130, "Device in X"=w131) -> ("Device out Y"=w126:refnum<k24>, "Device out X"=w127:refnum<k24>)  [unwired: 8 in]
          n91 = call "move-vector.vi"("GetPOS Y"=w111, "GetPOS X"=w112, "Device in Y"=w126, "X-Y"=w129, "Distance"=0.05, "Device in X"=w127) -> ("Device out Y"=w122:refnum<k24>, "Device out X"=w123:refnum<k24>)  [unwired: 4 in]
          n92 = Negate(x=0.1 ("Distance")) -> (-x=w121:dbl)
          n93 = call "move-vector.vi"("GetPOS Y"=w111, "GetPOS X"=w112, "Device in Y"=w122, "X-Y"=w125, "Distance"=w121, "Device in X"=w123) -> ("Device out Y"=w117:refnum<k24>, "Device out X"=w118:refnum<k24>)  [unwired: 4 in]
          n94 = call "move-vector.vi"("GetPOS Y"=w111, "GetPOS X"=w112, "Device in Y"=w117, "X-Y"=w120, "Distance"=0.05, "Device in X"=w118) -> ("Device out Y"=w113:refnum<k24>, "Device out X"=w114:refnum<k24>)  [unwired: 4 in]
          n95 = call "move-vector.vi"("GetPOS Y"=w111, "GetPOS X"=w112, "Device in Y"=w113, "X-Y"=w115, "Distance"=0.05, "Device in X"=w114) -> ("Device out Y"=w109:refnum<k24>, "Device out X"=w110:refnum<k24>)  [unwired: 4 in]
        }
        frame Enabled {
        }
      }
      n96 = disable-structure shown="Enabled" {
        disable-tunnel: [w180 w189] -> w93
        disable-tunnel: [w179 w188] -> w92
        disable-tunnel: w83 -> [w175 _]
        disable-tunnel: w82 -> [w174 _]
        disable-tunnel: w81 -> [w173 w189]
        disable-tunnel: w80 -> [w172 w188]
        frame Disabled {
          n97 = call "circuits-resistor-2.vi"("Invert X"=TRUE, "L3"=0.1, "L2"=0.05, "Swap-XY"=TRUE, "L1"=0.05, "Device in Y"=w172, "GetPOS Y"=w174, "GetPOS X"=w175, "Device in X"=w173) -> ("Device out Y"=w178:refnum<k24>, "Device out X"=w181:refnum<k24>)  [unwired: 1 in]
          n98 = call "circuits-resistor-2.vi"("Invert X"=TRUE ("Invert Y"), "L3"=0.1, "L2"=0.05, "Swap-XY"=TRUE, "L1"=0.05, "Device in Y"=w178, "GetPOS Y"=w174, "GetPOS X"=w175, "Device in X"=w181) -> ("Device out Y"=w179:refnum<k24>, "Device out X"=w180:refnum<k24>)  [unwired: 1 in]
        }
        frame Enabled {
        }
      }
      n99 = disable-structure shown="Enabled" {
        disable-tunnel: [w313 w317] -> w105
        disable-tunnel: [w312 w316] -> w104
        disable-tunnel: _ -> [w311 _]
        disable-tunnel: _ -> [w310 _]
        disable-tunnel: w93 -> [w309 w317]
        disable-tunnel: w92 -> [w308 w316]
        frame Disabled {
          n100 = call "circuits-resistor.vi"("L2"=0.025, "L1"=0.05, "Device in Y"=w308, "GetPOS Y"=w310, "GetPOS X"=w311, "Device in X"=w309) -> ("Device out Y"=w312:refnum<k24>, "Device out X"=w313:refnum<k24>)  [unwired: 4 in]
        }
        frame Enabled {
        }
      }
      n101 = disable-structure shown="Enabled" {
        disable-tunnel: w105 -> [w217 _]
        disable-tunnel: w104 -> [w216 _]
        disable-tunnel: w83 -> [w191 _]
        disable-tunnel: w82 -> [w190 _]
        frame Disabled {
          w199 = u16 0 items=["X", "Y"] ("X-Y")
          w205 = u16 1 items=["X", "Y"] ("X-Y")
          # "Fecha Shutter"
          # "Abre Shutter"
          n102 = call "circuits-capacitor.vi"("Invert Y"=TRUE, "L2"=0.025, "L3"=0.1, "Swap-XY"=TRUE, "L1"=0.1, "Device in Y"=w216, "GetPOS Y"=w190, "GetPOS X"=w191, "Device in X"=w217) -> ("Device out Y"=w209:refnum<k24>, "Device out X"=w210:refnum<k24>)  [unwired: 1 in]
          n103 = call "circuits-gound.vi"("GetPOS Y"=w190, "L1"=0.0, "GetPOS X"=w191, "Device in Y"=w209, "Device in X"=w210) -> ("Device out Y"=w207:refnum<k24>, "Device out X"=w208:refnum<k24>)  [unwired: 5 in]
          n104 = call "move-vector.vi"("GetPOS Y"=w190, "GetPOS X"=w191, "Device in Y"=w207, "X-Y"=w205, "Distance"=0.25, "Device in X"=w208) -> ("Device out Y"=w203:refnum<k24>, "Device out X"=w204:refnum<k24>)  [unwired: 4 in]
          n105 = call "Thorlabs-Shutter-Toggle.vi"("Device in Y"=w203, "Device in X"=w204) -> ("Device out Y"=w201:refnum<k24>, "Device out X"=w202:refnum<k24>)  [unwired: 8 in]
          n106 = call "move-vector.vi"("GetPOS Y"=w190, "GetPOS X"=w191, "Device in Y"=w201, "X-Y"=w199, "Distance"=0.1, "Device in X"=w202) -> ("Device out Y"=w197:refnum<k24>, "Device out X"=w198:refnum<k24>)  [unwired: 4 in]
          n107 = call "circuits-terminal.vi"("Density"=0.005, "GetPOS Y"=w190, "Diension"=0.1, "GetPOS X"=w191, "Device in Y"=w197, "Device in X"=w198) -> ("Device out Y"=w195:refnum<k24>, "Device out X"=w196:refnum<k24>)  [unwired: 4 in]
          n108 = call "Thorlabs-Shutter-Toggle.vi"("Device in Y"=w195, "Device in X"=w196) -> ()  [unwired: 8 in, 2 out]
        }
        frame Enabled {
        }
      }
    }
    frame #1 {
      w327 = FALSE
      n109 = local read ".NET Refnum out 2"() -> (w328:refnum<k24>)
      n110 = local read ".NET Refnum out 1"() -> (w329:refnum<k24>)
      n111 = local write "Stop Button"(FALSE ("Stop Button")) -> ()
      n112 = property on="Iniciar" class="Bool (strict)"("DisabledEnum"=T1."Disabled and Grayed Out" ("Disabled")) -> ()  [unwired: 2 in, 2 out]
      n113 = call "closeMotor.vi"(".NET Refnum in"=w329) -> ()  [unwired: 2 in]
      n114 = local write "Motor 2"(w327) -> ()
      n115 = local write "Motor 1"(w327) -> ()
      n116 = call "closeMotor.vi"(".NET Refnum in"=w328) -> ()  [unwired: 2 in]
      "stop cronometro" <- TRUE ("stop cronometro")
    }
  }
  n117 = case shown="True" w1 {
    frame False {
    }
    frame True {
      # "Graph"
      n118 = flat-sequence {
        frame #0 {
          w330 = 0.0
          n119 = local write "GetPOS Y"(w330) -> ()
          n120 = local write "GetPOS X"(w330) -> ()
        }
        frame #1 {
          n121 = while {
            stop <- w331 stop-if-true
            n122 = flat-sequence {
              frame #0 {
                n123 = local read "GetPOS X"() -> (w336:dbl)
                n124 = local read "GetPOS Y"() -> (w335:dbl)
                n125 = local read "Graph X"() -> (w338:dbl[])
                n126 = local read "Graph Y"() -> (w333:dbl[])
                n127 = Build Array (concatenate)(w338, w336) -> (w337:dbl[])
                n128 = local write "Graph X"(w337) -> ()
                n129 = Build Array (concatenate)(w333, w335) -> (w334:dbl[])
                n130 = local write "Graph Y"(w334) -> ()
              }
              frame #1 {
                n131 = Array Subset(array="Graph Y", index=3) -> (w339:dbl[])  [unwired: 1 in]
                n132 = Array Subset(array="Graph X", index=3) -> (w342:dbl[])  [unwired: 1 in]
                n133 = Bundle(w342, w339) -> (→"XY Graph":cluster{dbl[], dbl[]})  [unwired: 1 in]
              }
            }
            n134 = local read "stop cronometro"() -> (w331:bool)
            n135 = Wait (ms)(milliseconds to wait=u32 100) -> ()  [unwired: 1 out]
          }
        }
      }
    }
  }
  n136 = case shown="True" w1 {
    frame False {
    }
    frame True {
      # "Shutter Control"
      n137 = flat-sequence {
        tunnel: [w351] -> w349
        tunnel: [w350] -> w348
        tunnel: w349 -> [w369]
        tunnel: w348 -> [w366]
        tunnel: [w368] -> w347
        tunnel: [w367] -> w346
        tunnel: w347 -> [w387]
        tunnel: w346 -> [w386]
        frame #0 {
          w361 = u16 0 items=["None", "Odd", "Even", "Mark", "Space"] ("parity")
          w358 = u16 10 items=["1.0"=10, "1.5"=15, "2.0"=20] ("stop bits")
          w357 = u16 0 items=["None"=0, "XON/XOFF"=1, "RTS/CTS"=2, "DTR/DSR"=4] ("flow control")
          w359 = FALSE  # Enable Termination Char (T)
          w360 = u32 10000  # timeout (10sec)
          # "Configura a porta serial usada pela Shutter"
          # "Configure Serial port (baud rate,\ndata bits, parity, stop bits and flow control)."
          # "Seleciona o \nmode de operação\nda Shutter"
          # "Abre a Shutter por um longo\nperíodo de tempo"
          n138 = call-poly "VISA Configure Serial Port"("VISA resource name"=refnum<visa-resource-name> "COM3", "timeout (10sec)"=w360, "Enable Termination\nChar (T)"=w359, "baud rate (9600)"=u32 9600 ("baud rate"), "data bits (8)"=u16 8 ("data bits"), "parity (0:none)"=w361, "stop bits (10: 1 bit)"=w358, "flow control (0:none)"=w357) -> ("VISA resource name out"=w355:refnum<visa-resource-name>, "error out"=w354:errorcluster)  [unwired: 6 in]
          n139 = VISA Write(VISA resource name=w355, write buffer="mode=3\r", error in (no error)=w354) -> (VISA resource name out=w353:refnum<visa-resource-name>, error out=w352:errorcluster)  [unwired: 1 out]
          n140 = VISA Write(VISA resource name=w353, write buffer="open=900000\r", error in (no error)=w352) -> (VISA resource name out=w351:refnum<visa-resource-name>, error out=w350:errorcluster)  [unwired: 1 out]
        }
        frame #1 {
          n141 = while {
            tunnel: w369 -> [w376]
            tunnel: [w375] -> w368
            tunnel: [w374] -> w367
            tunnel: w366 -> [w373]
            stop <- w370 stop-if-true
            n142 = global read "motorsGlobalVar.vi" "Shutter toggle"() -> (w372:bool)
            n143 = Wait (ms)(milliseconds to wait=u32 1) -> ()  [unwired: 1 out]
            n144 = case shown="False" w372 {
              tunnel: w376 -> [w378 w383]
              tunnel: [w378 w382] -> w375
              tunnel: [w377 w381] -> w374
              tunnel: w373 -> [w377 w380]
              frame False {
              }
              frame True {
                n145 = global write "motorsGlobalVar.vi" "Shutter toggle"(FALSE ("Shutter toggle")) -> ()
                n146 = VISA Write(VISA resource name=w383, write buffer="ens\r", error in (no error)=w380) -> (VISA resource name out=w382:refnum<visa-resource-name>, error out=w381:errorcluster)  [unwired: 1 out]
              }
            }
            n147 = local read "stop cronometro"() -> (w370:bool)
          }
        }
        frame #2 {
          n148 = VISA Close(VISA resource name=w387, error in (no error)=w386) -> (error out=w385:errorcluster)
          n149 = call <vilib>:"Clear Errors.vi"("error in (no error)"=w385) -> ()  [unwired: 5 in, 2 out]
        }
      }
    }
  }
